vi "Decide Procedure Next State.vi"(11 "Prev State":T1=enum."Warm Up") -> (1 "ResetEyeTrack":bool, 3 "New State":T1=enum."Warm Up")   [LabVIEW 2015]
uses:
  Controls/BELKIN RT State.ctl
  Stream/LP Globals.vi
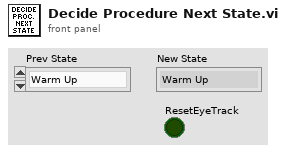
[diagram p1: front panel]
types:
  T1 = typedef "BELKIN RT State.ctl" = enum16{"Initialize", "BIT", "Warm Up", "Eye Location", "Find Limbus", "Eye Track", "Fire", "Treatment Complete", "Shut Down", "Error"}
  T2 = typedef "Command Typedef.ctl" = cluster{"CMD":T1, "Data":variant}
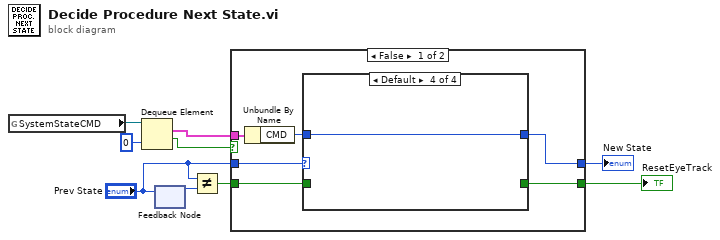
[diagram p0: block diagram]
diagram:
  n1 = global read "LP Globals.vi" "SystemStateCMD"() -> (w5:refnum<queue>)
  n2 = Dequeue Element(queue=w5, timeout in ms (-1)=0) -> (element=w7:T2, timed out?=w8:bool)  [unwired: 1 in, 2 out]
  n3 = feedback-in #1("Prev State") -> ()
  n4 = feedback #1() -> (w4:T1)  [unwired: 1 in]
  n5 = Not Equal?(x="Prev State", y=w4) -> (x != y?=w2:bool)
  n6 = case shown="False" w8 {
    tunnel: "Prev State" -> [w15 w26]
    tunnel: w7 -> [w14 _]
    tunnel: [w12 w26] -> w9
    tunnel: w2 -> [w11 w25]
    tunnel: [w10 w25] -> w1
    frame False {
      n7 = Unbundle By Name(w14) -> ("CMD"=w13:T1)
      n8 = case shown="Default" w15 {
        selector: w15 -> [w16 _ _ _]
        tunnel: [w17 w21 w23 w24] -> w12
        tunnel: w13 -> [w18 w21 w23 w24]
        tunnel: [_ _ w22 _] -> w10
        tunnel: w11 -> [_ _ w22 _]
        frame "Warm Up" {
          n9 = case shown="\"Eye Location\"" w18 {
            selector: w18 -> [_ w20]
            tunnel: [w19 w20] -> w17
            tunnel: w16 -> [w19 _]
            frame Default {
            }
            frame "Eye Location" {
            }
          }
        }
        frame "Eye Location" {
        }
        frame "Find Limbus" {
        }
        frame Default {
        }
      }
    }
    frame True {
    }
  }
  "New State" <- w9
  "ResetEyeTrack" <- w1
